vi "Scan For App Projects.vi"(8 "error in":errorcluster, 10 "Init?":bool, 11 "Projects Ref":refnum<vi>) -> (0 "error out":errorcluster)   [LabVIEW 2019, in "Panther Dashboard.lvlib"]
uses:
  Panther Dashboard.lvlib
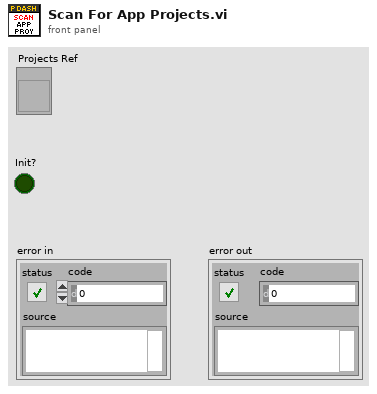
[diagram p1: front panel]
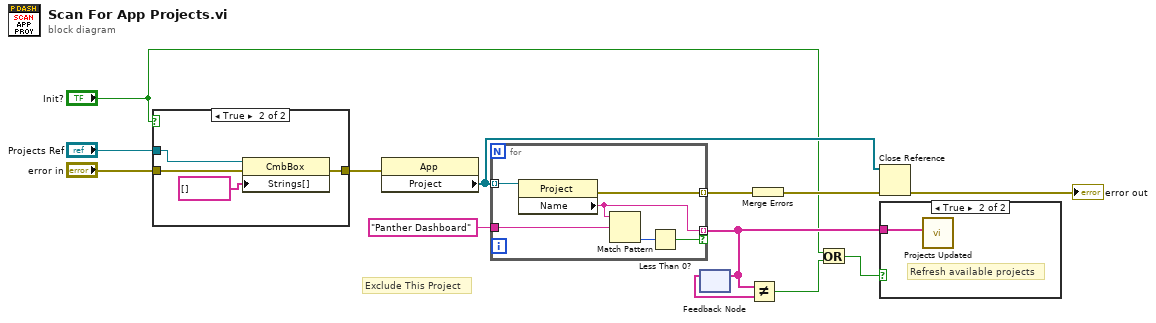
[diagram p0: block diagram]
diagram:
  # "Exclude This Project"
  n1 = case shown="True" "Init?" {
    tunnel: "Projects Ref" -> [_ w16]
    tunnel: "error in" -> [w14 w18]
    tunnel: [w14 w17] -> w10
    frame False {
    }
    frame True {
      n2 = property class="CmbBox"(reference=w16, error in=w18, "Strings[]"=string[] []) -> (error out=w17:errorcluster)  [unwired: 1 out]
    }
  }
  n3 = property class="App"(error in=w10) -> ("Project"=w8:refnum<vi>[])  [unwired: 1 in, 2 out]
  n4 = for {
    tunnel: w8 -> [w19] mode=indexing
    tunnel: [w23] -> w5 mode=indexing if=w20
    tunnel: "Panther Dashboard" -> [w22]
    tunnel: [w24] -> w7 mode=indexing
    n5 = property class="Project"(reference=w19) -> (error out=w24:errorcluster, "Name"=w23:string)  [unwired: 1 in, 1 out]
    n6 = Match Pattern(string=w23, regular expression=w22) -> (offset past match=w21:i32)  [unwired: 1 in, 3 out]
    n7 = Less Than 0?(x=w21) -> (x < 0?=w20:bool)
  }
  n8 = feedback-in #1(w5) -> ()
  n9 = feedback #1() -> (w6:string[])  [unwired: 1 in]
  n10 = Not Equal?(x=w5, y=w6) -> (x != y?=w4:bool)
  n11 = Merge Errors(w7) -> (w12:errorcluster)
  n12 = Or(x="Init?", y=w4) -> (x .or. y?=w2:bool)
  n13 = Close Reference(reference=w8, error in (no error)=w12) -> (error out=→"error out":errorcluster)
  n14 = case shown="True" w2 {
    tunnel: w5 -> [_ w25]
    frame False {
    }
    frame True {
      # "Refresh available projects"
      n15 = call "Projects Updated.vi"("Projects"=w25) -> ()  [unwired: 10 in, 1 out]
    }
  }
